vi "Query-Limits.vi"(6 "error in (no error)":errorcluster, 7 "Output channel":T1, 8 "VISA resource name":refnum<visa-resource-name>) -> (0 "error out":errorcluster, 2 "Recalled minimum / V":dbl, 3 "Recalled maximum / V":dbl, 5 "VISA resource name out":refnum<visa-resource-name>)   [LabVIEW 2015, in "YbTempCtrl.lvlib"]
doc: "Queries the current output limits"
uses:
  YbTempCtrl.lvlib
  Typedefs/OutputChannelTypedef.ctl
panel:
  out "read buffer":string
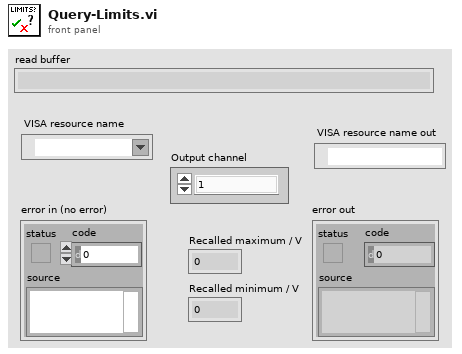
[diagram p1: front panel]
types:
  T1 = typedef "YbTempCtrl.lvlib/OutputChannelTypedef.ctl" = enum16{"1", "2", "3", "4", "BPA", "BPB"}
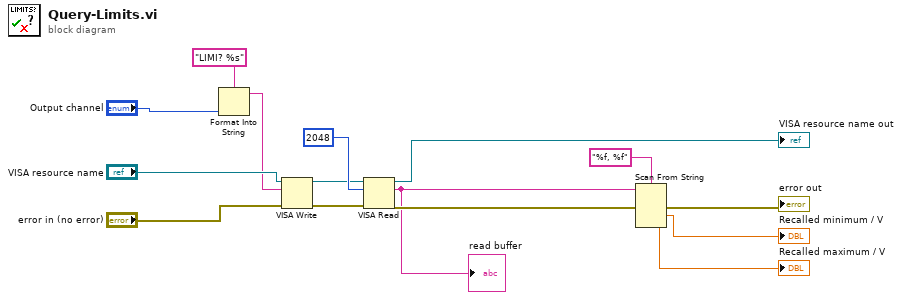
[diagram p0: block diagram]
diagram:
  n1 = Format Into String(format string="LIMI? %s" ("write buffer"), "Output channel") -> (resulting string=w8:string)  [unwired: 2 in, 1 out]
  n2 = VISA Write(VISA resource name="VISA resource name", write buffer=w8, error in (no error)="error in (no error)") -> (VISA resource name out=w7:refnum<visa-resource-name>, error out=w6:errorcluster)  [unwired: 1 out]
  n3 = VISA Read(VISA resource name=w7, byte count=u32 2048, error in (no error)=w6) -> (VISA resource name out=→"VISA resource name out":refnum<visa-resource-name>, read buffer=w4:string, error out=w10:errorcluster)  [unwired: 1 out]
  "read buffer" <- w4
  n4 = Scan From String(format string="%f, %f", input string=w4, error in=w10) -> (error out=→"error out":errorcluster, output 1=→"Recalled minimum / V":dbl, output 2=→"Recalled maximum / V":dbl)  [unwired: 3 in, 2 out]
